vi "pid_pi_p_Process reaction_Method.vi"() -> ()   [LabVIEW 2021]
uses:
  <vilib>/picture/cartesn2.llb/XY Plot Type.ctl
panel:
  in  "XY plot cosmetics":T2={"plot color"=16776960, "XY plot type"=enum."connected points", "baseline"=0.0} {"baseline" format="%0.2f"}
  out "new picture":picture
  in  "Controller_type":string(combo)="PID"
  out "appended array":dbl[](array[numeric])=[nan, 0.0, 0.0]
  out "L":dbl
  out "T":dbl=nan
  out "k":dbl
  in  "t_array":dbl[](array[numeric])=[0.0, 0.5, 1.0, 1.5, 2.0, 2.5, 3.0, 3.5, 4.0, 4.5, 5.0, 5.5, 6.0, 7.0, 7.0]
  in  "u_array":dbl[](array[numeric])=[1.0, 0.0, 0.0, 0.0, 0.0, 0.0, 0.0, 0.0, 0.0, 0.0, 0.0, 0.0, 0.0, 0.0, 0.0, 0.0, -5000.0]
  in  "y_array":dbl[](array[numeric])=[0.0, 0.02, 0.05, 0.16, 0.28, 0.42, 0.58, 0.7, 0.8, 0.86, 0.92, 0.95, 0.97, 0.98]
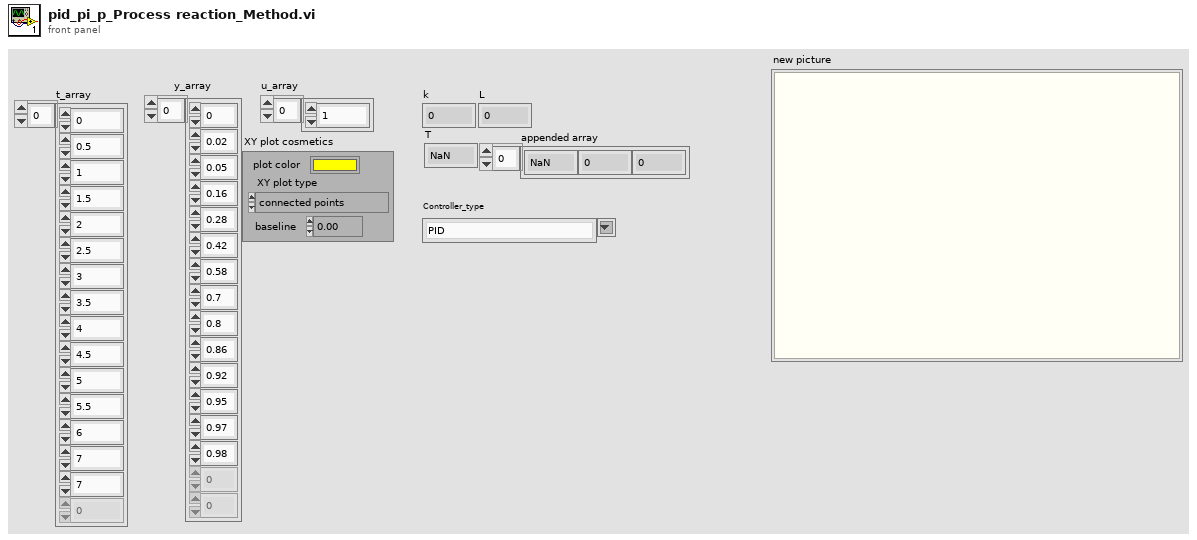
[diagram p1: front panel]
types:
  T1 = typedef "XY Plot Type.ctl" = enum16{"points", "squares", "circles", "connected points", "connected squares", "connected circles", "comb plot", "sized scatter plot", "sized-colored scatter plot", "min-max lines"}
  T2 = cluster{"plot color":u32, "XY plot type":T1, "baseline":dbl}
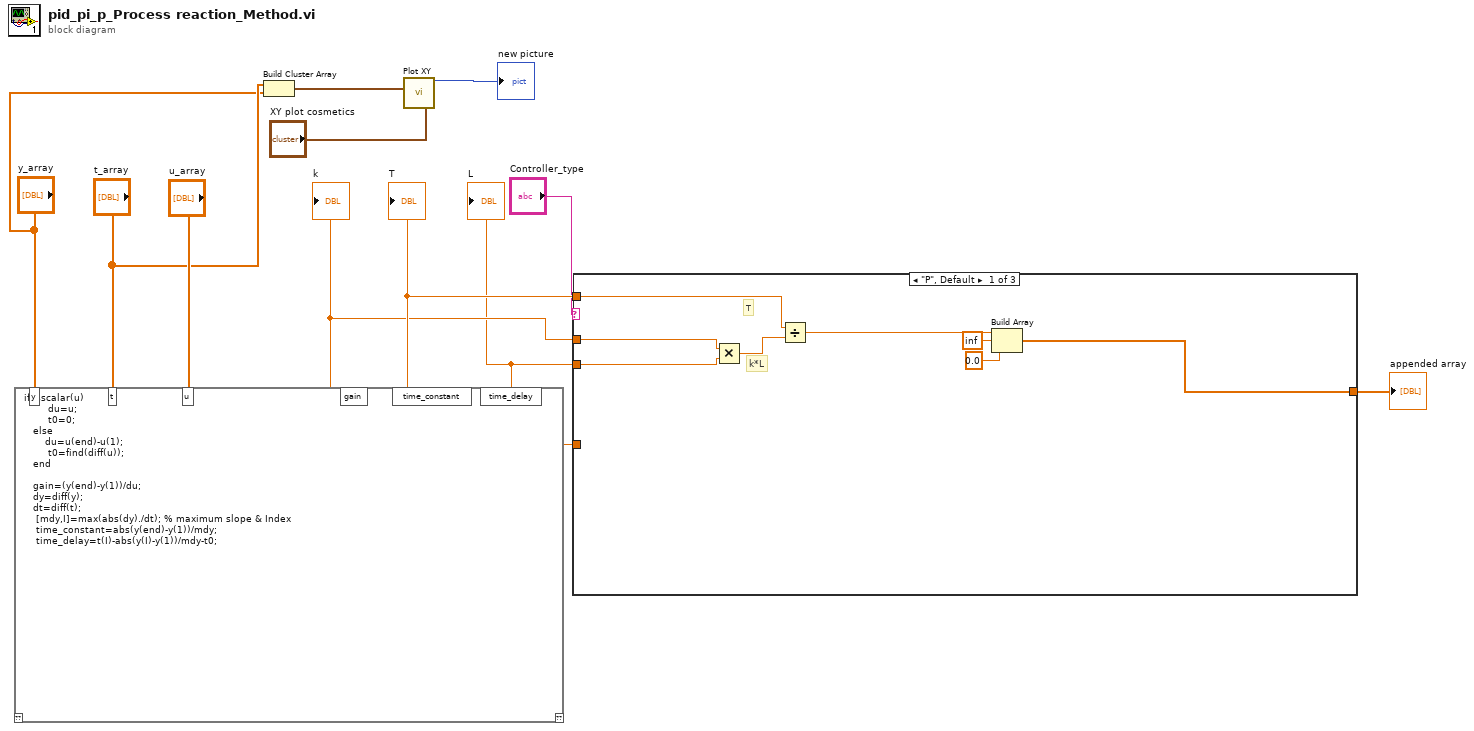
[diagram p0: block diagram]
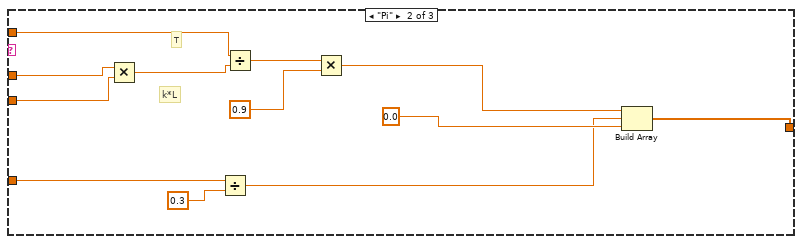
[diagram p2: hidden frame]
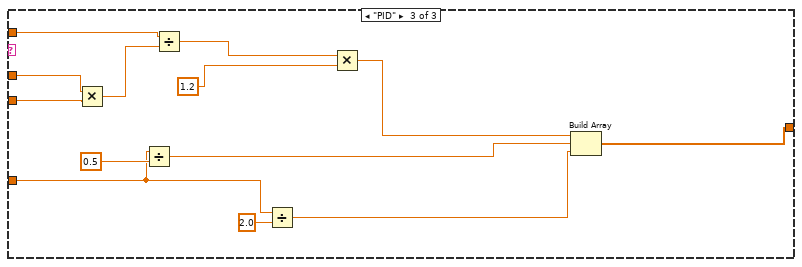
[diagram p3: hidden frame]
diagram:
  n1 = script code="if isscalar(u)\n        du=u;\n        t0=0;\n   else\n       du=u(end)-u(1);\n        t0=find(diff(u));\n   end\n\n   gain=(y(end)-y(1))/du;\n   dy=diff(y);\n   dt=diff(t);\n    [mdy,I]=max(abs(dy)./dt); % maximum slope & Index\n    time_constant=abs(y(end)-y(1))/mdy;\n    time_delay=t(I)-abs(y(I)-y(1))/mdy-t0;"("y"="y_array", "u"="u_array", "t"="t_array") -> ("gain"=w9:dbl, "time_constant"=w10:dbl, "time_delay"=w8:dbl)  [unwired: 1 in, 1 out]
  "k" <- w9
  "T" <- w10
  "L" <- w8
  n2 = Build Cluster Array("t_array", "y_array") -> (w5:cluster{dbl, dbl}[])
  n3 = call <vilib>:"Plot XY.vi"("data"=w5, "XY plot cosmetics"="XY plot cosmetics") -> ("new picture"=→"new picture":picture)  [unwired: 13 in]
  n4 = case shown="\"P\", Default" "Controller_type" {
    tunnel: w10 -> [w15 w24 w35]
    tunnel: w9 -> [w16 w23 w34]
    tunnel: w8 -> [w17 w22 w33]
    tunnel: w8 -> [_ w21 w32]
    tunnel: [w14 w20 w36] -> w7
    frame "P", Default {
      # "k*L"
      # "T"
      n5 = Multiply(x=w16, y=w17) -> (x*y=w19:dbl)
      n6 = Divide(x=w15, y=w19) -> (x/y=w18:dbl)
      n7 = Build Array(w18, inf ("element"), 0.0 ("element")) -> (w14:dbl[])
    }
    frame "Pi" {
      # "k*L"
      # "T"
      n8 = Multiply(x=w23, y=w22) -> (x*y=w31:dbl)
      n9 = Divide(x=w21, y=0.3) -> (x/y=w25:dbl)
      n10 = Divide(x=w24, y=w31) -> (x/y=w28:dbl)
      n11 = Multiply(x=w28, y=0.9) -> (x*y=w27:dbl)
      n12 = Build Array(w27, w25, 0.0 ("element")) -> (w20:dbl[])
    }
    frame "PID" {
      n13 = Multiply(x=w34, y=w33) -> (x*y=w44:dbl)
      n14 = Divide(x=w32, y=0.5) -> (x/y=w39:dbl)
      n15 = Divide(x=w35, y=w44) -> (x/y=w42:dbl)
      n16 = Divide(x=w32, y=2.0) -> (x/y=w37:dbl)
      n17 = Multiply(x=w42, y=1.2) -> (x*y=w41:dbl)
      n18 = Build Array(w41, w39, w37) -> (w36:dbl[])
    }
  }
  "appended array" <- w7
